vi "Get Property Values (String Property).vi"(1 "data type":string[](array[string]), 5 "property":T2 {"data type" items=["Unknown"=0, "String"=23, "I32"=3, "I64"=4, "DBL"=10, "Time stamp"=30]; "object type" items=["File", "Channel Group", "Channel"]}, 7 "result references":T1[](array[typedef]), 11 "error in (no error)":errorcluster) -> (6 "property values":string[](array[string]), 8 "result references out":T1[](array[typedef]), 15 "error out":errorcluster)   [LabVIEW 2020, in "NI_DataFinder.lvlib"]
doc: "Determines from the result references the values of a string property."
uses:
  <vilib>/DataFinder/NI_DataFinder.lvlib
  <vilib>/DataFinder/DataTypes/property.ctl
  <vilib>/DataFinder/DataTypes/object type.ctl
  <vilib>/DataFinder/DataTypes/data type.ctl
  <vilib>/userdefined/DFSearchResult.ctl
  <vilib>/userdefined/NI_DataFinder Controls.lvlib
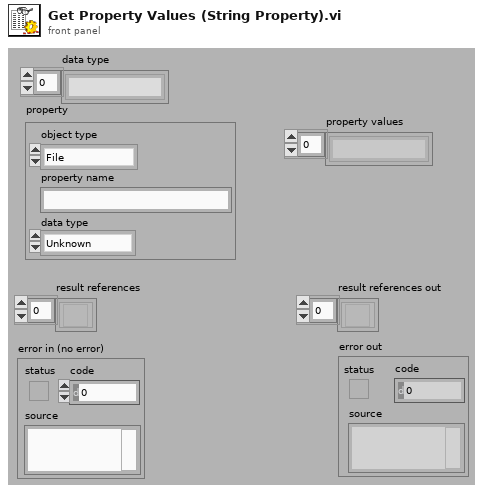
[diagram p1: front panel]
types:
  T1 = typedef "NI_DataFinder Controls.lvlib/DFSearchResult.ctl" = refnum<k20>
  T2 = typedef "NI_DataFinder.lvlib/property.ctl" = cluster{"object type":T3, "property name":string, "data type":T4}
  T3 = typedef "NI_DataFinder.lvlib/object type.ctl" = u16
  T4 = typedef "NI_DataFinder.lvlib/data type.ctl" = u16
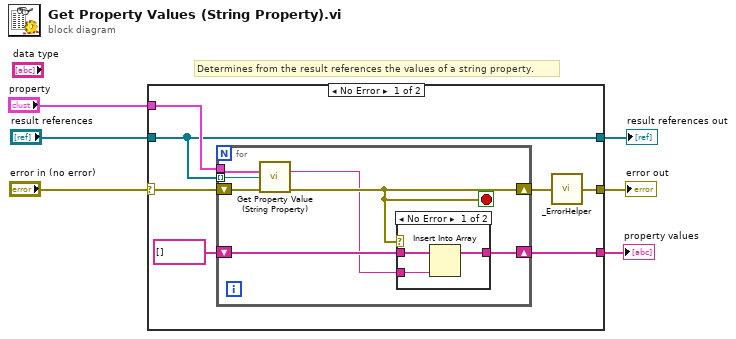
[diagram p0: block diagram]
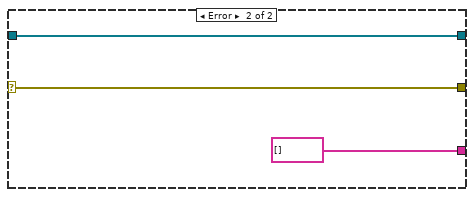
[diagram p3: hidden frame]
diagram:
  # "Determines from the result references the values of a string property."
  n1 = case shown="No Error" "error in (no error)" {
    selector: "error in (no error)" -> [w13 w27]
    tunnel: "property" -> [w12 _]
    tunnel: [w10 w27] -> w4
    tunnel: "result references" -> [w9 w26]
    tunnel: [w9 w26] -> w1
    tunnel: [w11 string[] []] -> w3
    frame No Error {
      n2 = for {
        tunnel: w9 -> [w16] mode=indexing
        tunnel: w12 -> [w15]
        shift-right: [w17] -> w8
        shift-left: w13 -> [w18]
        shift-right: [w20] -> w11
        shift-left: string[] [] -> [w19]
        stop <- w17 stop-if-true
        n3 = call <vilib>:"Get Property Value (String Property).vi"("property"=w15, "result reference"=w16, "error in (no error)"=w18) -> ("property value"=w14:string, "error out"=w17:errorcluster)  [unwired: 10 in, 1 out]
        n4 = case shown="No Error" w17 {
          tunnel: w19 -> [w23 w24]
          tunnel: w14 -> [w22 _]
          tunnel: [w21 w24] -> w20
          frame No Error {
            n5 = Insert Into Array(array=w23, new element=w22) -> (w21:string[])  [unwired: 1 in]
          }
          frame Error {
          }
        }
      }
      n6 = call <vilib>:"_ErrorHelper.vi"("error IO"=w8) -> ("error out"=w10:errorcluster)
    }
    frame Error {
    }
  }
  "error out" <- w4
  "result references out" <- w1
  "property values" <- w3
